vi "Calculate Sun Elevation from Position and Time.vi"(5 "Lat":dbl, 7 "Long":dbl, 11 "date time rec (UTC)":T1) -> (3 "Solar Elevation Angle":dbl)   [LabVIEW 2014, in "Solar Calculations.lvlib"]
uses:
  Solar Calculations.lvlib
  <vilib>/Utility/miscctls.llb/LVDateTimeRec.ctl
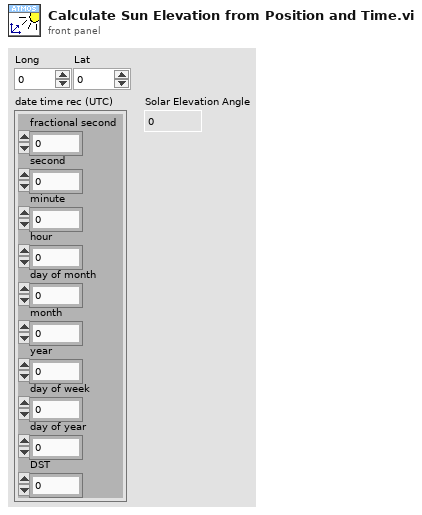
[diagram p1: front panel]
types:
  T1 = typedef "LVDateTimeRec.ctl" = cluster{"fractional second":dbl, "second":i32, "minute":i32, "hour":i32, "day of month":i32, "month":i32, "year":i32, "day of week":i32, "day of year":i32, "DST":i32}
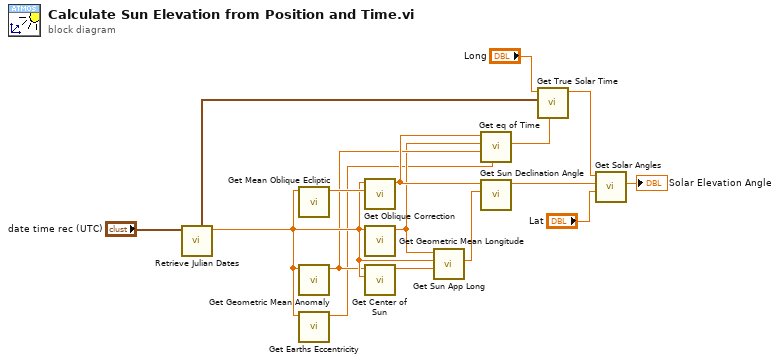
[diagram p0: block diagram]
diagram:
  n1 = call "Retrieve Julian Dates.vi"("Date Time (UTC)"="date time rec (UTC)") -> ("Julian Century"=w8:dbl, "Timestamp (local)"=w1:timestamp)  [unwired: 8 in, 1 out]
  n2 = call "Get Mean Oblique Ecliptic.vi"("Julian Century"=w8) -> ("Mean Obique Ecliptic Longitude"=w11:dbl)  [unwired: 10 in]
  n3 = call "Get Geometric Mean Anomaly.vi"("Julian Century"=w8) -> ("Mean Anomaly"=w7:dbl)  [unwired: 10 in]
  n4 = call "Get Earths Eccentricity.vi"("Julian Century"=w8) -> ("Eccentricity"=w5:dbl)  [unwired: 10 in]
  n5 = call "Get Oblique Correction.vi"("Mean Obique Ecliptic Longitude"=w11, "Julian Century"=w8) -> ("Oblique Correction (deg)"=w9:dbl)  [unwired: 9 in]
  n6 = call "Get Geometric Mean Longitude.vi"("Julian Century"=w8) -> ("Geometric Mean Longitude"=w6:dbl)  [unwired: 10 in]
  n7 = call "Get Center of Sun.vi"("Julian Century"=w8, "Geometric Mean Anomaly"=w7) -> ("Sun Eq of Ctr"=w12:dbl)  [unwired: 9 in]
  n8 = call "Get Sun App Long.vi"("Sun Eq of Ctr"=w12, "Julian Century"=w8, "Geometric Mean Longitude"=w6) -> ("Sun App Long (deg)"=w10:dbl)  [unwired: 7 in, 1 out]
  n9 = call "Get eq of Time.vi"("Eccentricity"=w5, "Mean Anomaly"=w7, "Geometric Mean Longitude"=w6, "Oblique Correction (deg)"=w9) -> ("Eq of Time (min)"=w4:dbl)  [unwired: 6 in, 1 out]
  n10 = call "Get Sun Declination Angle.vi"("Sun App Long (deg)"=w10, "Oblique Correction (deg)"=w9) -> ("Numeric"=w2:dbl)  [unwired: 9 in]
  n11 = call "Get True Solar Time.vi"("Eq of Time (min)"=w4, "time (utc)"=w1, "Long"="Long") -> ("TST (min)"=w3:dbl)  [unwired: 8 in]
  n12 = call "Get Solar Angles.vi"("lattitude"="Lat", "Numeric 3"=w2, "TST (min)"=w3) -> ("Solar Elevation Angle (deg)"=→"Solar Elevation Angle":dbl)  [unwired: 6 in, 2 out]
